vi "Close Instrument.vi"(8 "error in (no error)":errorcluster, 11 "Instrument in":refnum<class "Instrument.lvclass">) -> (0 "error out":errorcluster, 3 "Instrument out":refnum<class "Instrument.lvclass">)   [LabVIEW 2017, in "Instrument.lvlib" / "Instrument.lvclass"]
doc: "Closes an instrument and clears out any internal references to the physical connection address [e.g. close COM port, uninitialize GPIB]"
uses:
  Instrument.lvclass
  Instrument.lvclass/Instrument.ctl
  Properties/Instrument Properties.lvclass/Instrument Properties.ctl
  Properties/Instrument Properties.lvclass
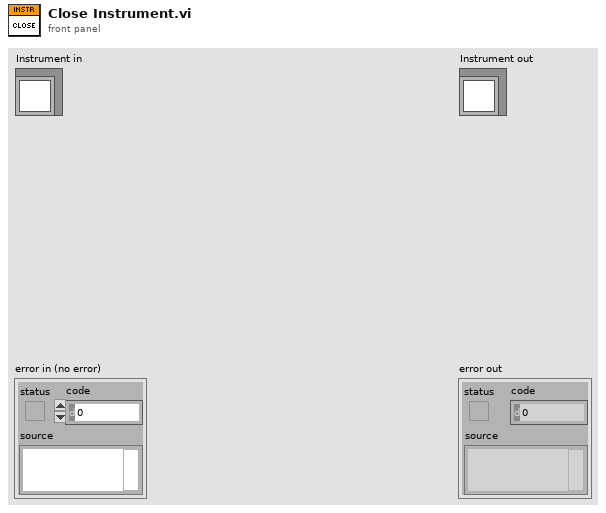
[diagram p1: front panel]
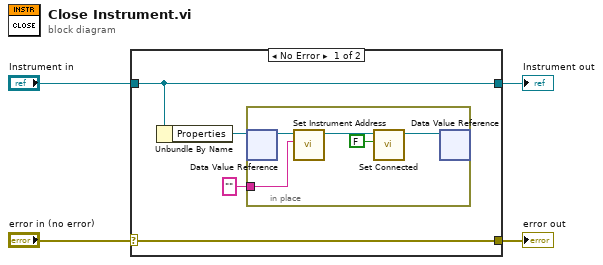
[diagram p0: block diagram]
diagram:
  n1 = case shown="No Error" "error in (no error)" {
    selector: "error in (no error)" -> [w8 w15]
    tunnel: [w8 w15] -> w3
    tunnel: [w7 w14] -> w1
    tunnel: "Instrument in" -> [w7 w14]
    frame No Error {
      n2 = Unbundle By Name(w7) -> ("Properties"=w6:refnum<data-value>)
      n3 = in-place {
        in-place-border: "" -> [w12]
        n4 = in-place-dvr #1(w6) -> (w13:refnum<class "Instrument Properties.lvclass">)  [unwired: 1 out]
        n5 = call-dynamic "Set Instrument Address.vi"("Instrument Address"=w12, "Instrument Properties in"=w13) -> ("Instrument Properties out"=w11:refnum<class "Instrument Properties.lvclass">)  [unwired: 8 in, 1 out]
        n6 = call "Set Connected.vi"("Connected"=FALSE, "Instrument Properties in"=w11) -> ("Instrument Properties out"=w10:refnum<class "Instrument Properties.lvclass">)  [unwired: 8 in, 1 out]
        n7 = in-place-dvr #1(w10) -> ()  [unwired: 2 out]
      }
    }
    frame Error {
    }
  }
  "error out" <- w3
  "Instrument out" <- w1
